vi "Elapsed Times.vi"(3 "Call Name":string) -> (1 "Timings":cluster{"Call Name":string, "Delta (ms)":u32}[](array[cluster]))   [LabVIEW 2017]
doc: "This VI will display the time between subsequent calls. Place it in a loop such as TeleOp, or a Controller, and it will measure and display the time between calls of a particular site."
panel:
  out "Call Name 2":string
  in  "Index":i32
  out "Waveform Chart":u32(graph)
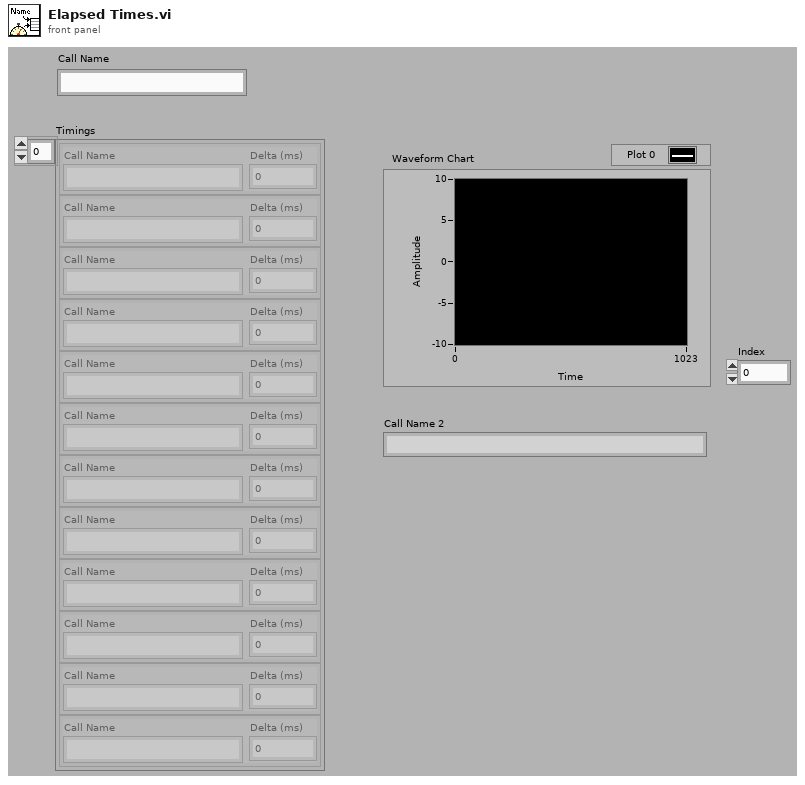
[diagram p1: front panel]
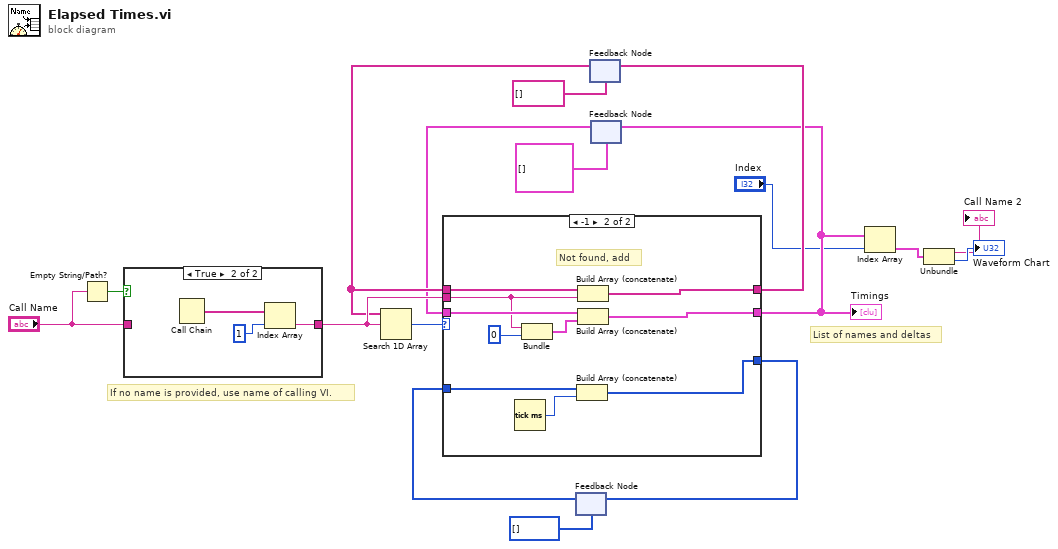
[diagram p0: block diagram]
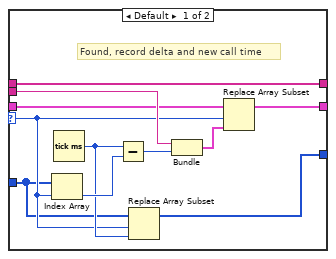
[diagram p2: hidden frame]
diagram:
  # "List of names and deltas"
  # "If no name is provided, use name of calling VI."
  n1 = Empty String/Path?(string/path="Call Name") -> (empty?=w17:bool)
  n2 = case shown="True" w17 {
    tunnel: "Call Name" -> [w18 _]
    tunnel: [w18 w21] -> w14
    frame False {
    }
    frame True {
      n3 = Call Chain() -> (call chain=w20:string[])
      n4 = Index Array(array=w20, index=1 ("millisecond timer value")) -> (element=w21:string)
    }
  }
  n5 = feedback #1(u32[] []) -> (w9:u32[])
  n6 = feedback #2(string[] []) -> (w12:string[])
  n7 = Search 1D Array(1D array=w12, element=w14) -> (index of element=w15:i32)  [unwired: 1 out]
  n8 = feedback #3(cluster{"Name":string, u32}[] []) -> (w7:cluster{"Call Name":string, u32}[])
  n9 = case shown="-1" w15 {
    selector: w15 -> [w24 _]
    tunnel: w14 -> [w30 w35]
    tunnel: [w28 w41] -> w13
    tunnel: w12 -> [w28 w40]
    tunnel: [w22 w39] -> w10
    tunnel: w9 -> [w23 w38]
    tunnel: [w27 w33] -> w5
    tunnel: w7 -> [w26 w37]
    frame Default {
      # "Found, record delta and new call time"
      n10 = Index Array(array=w23, index=w24) -> (element=w32:u32)
      n11 = Tick Count (ms)() -> (millisecond timer value=w25:u32)
      n12 = Subtract(x=w25, y=w32) -> (x-y=w31:u32)
      n13 = Replace Array Subset(array=w23, new element=w25, index=w24) -> (w22:u32[])
      n14 = Bundle("Call Name"=w30, w31) -> (w29:cluster{"Call Name":string, u32})  [unwired: 1 out]
      n15 = Replace Array Subset(array=w26, new element=w29, index=w24) -> (w27:cluster{"Call Name":string, u32}[])
    }
    frame -1 {
      # "Not found, add"
      n16 = Tick Count (ms)() -> (millisecond timer value=w42:u32)
      n17 = Bundle("Call Name"=w35, 0) -> (w34:cluster{"Call Name":string, i32})  [unwired: 1 out]
      n18 = Build Array (concatenate)(w38, w42) -> (w39:u32[])
      n19 = Build Array (concatenate)(w40, w35) -> (w41:string[])
      n20 = Build Array (concatenate)(w37, w34) -> (w33:cluster{"Call Name":string, u32}[])
    }
  }
  "Timings" <- w5
  n21 = feedback-in #1(w10) -> ()
  n22 = feedback-in #2(w13) -> ()
  n23 = feedback-in #3(w5) -> ()
  n24 = Index Array(array=w5, index="Index") -> (element=w3:cluster{"Call Name":string, u32})
  n25 = Unbundle(w3) -> ("Call Name"=→"Call Name 2":string, →"Waveform Chart":u32)
